vi "Day 2 Puzzle 2.vi"() -> ()   [LabVIEW 2021]
uses:
  <vilib>/Utility/file.llb/Read Delimited Spreadsheet (string).vi
panel:
  out "Sum":i32
  out "Outcomes":i32[](array[numeric])
  in  "Path":path
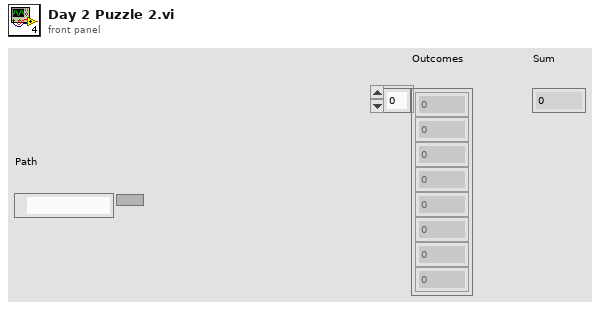
[diagram p1: front panel]
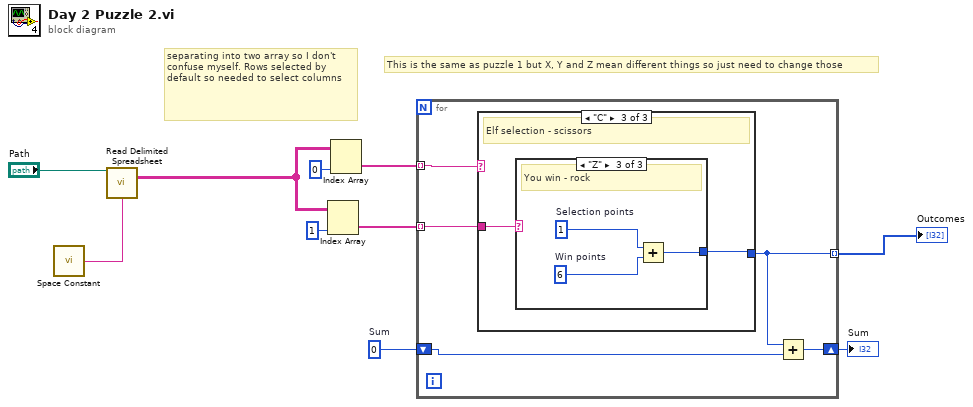
[diagram p0: block diagram]
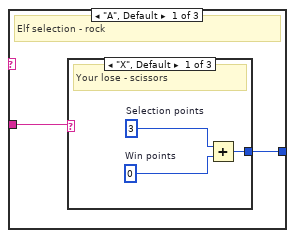
[diagram p2: hidden frame]
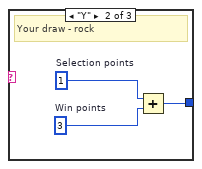
[diagram p3: hidden frame]
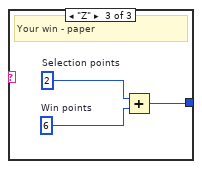
[diagram p4: hidden frame]
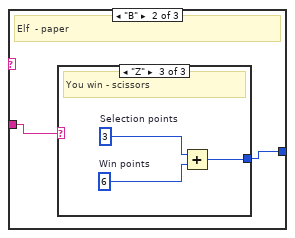
[diagram p5: hidden frame]
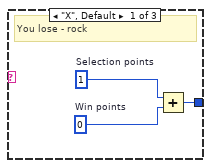
[diagram p6: hidden frame]
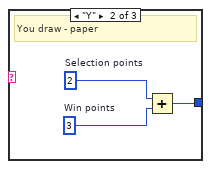
[diagram p7: hidden frame]
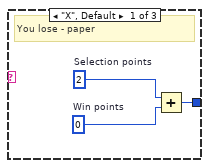
[diagram p8: hidden frame]
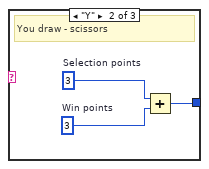
[diagram p9: hidden frame]
diagram:
  w2 = 0  # Sum
  # "This is the same as puzzle 1 but X, Y and Z mean different things so just need to change those"
  # "separating into two array so I don't confuse myself. Rows selected by default so needed to select columns"
  n1 = call <vilib>:"Space Constant.vi"() -> ("String"=w9:string)
  n2 = call-poly <vilib>:"Read Delimited Spreadsheet.vi"("file path (dialog if empty)"="Path", "delimiter (\\t)"=w9) -> ("all rows"=w8:string[][])  [unwired: 8 in, 5 out]
  n3 = Index Array(array=w8, index (col)=1 ("disabled index (col)")) -> (element=w6:string[])  [unwired: 1 in]
  n4 = Index Array(array=w8, index (col)=0 ("disabled index (col)")) -> (element=w7:string[])  [unwired: 1 in]
  n5 = for {
    tunnel: w7 -> [w15] mode=indexing
    tunnel: w6 -> [w14] mode=indexing
    tunnel: [w12] -> w3 mode=indexing
    shift-right: [w13] -> w1
    shift-left: w2 -> [w11]
    n6 = case shown="\"C\"" w15 {
      tunnel: w14 -> [w17 w27 w39]
      tunnel: [w16 w28 w38] -> w12
      frame "A", Default {
        # "Elf selection - rock"
        n7 = case shown="\"X\", Default" w17 {
          tunnel: [w18 w21 w24] -> w16
          frame "X", Default {
            w20 = 0  # Win points
            w19 = 3  # Selection points
            # "Your lose - scissors"
            n8 = Add(x=w19, y=w20) -> (x+y=w18:i32)
          }
          frame "Y" {
            w23 = 3  # Win points
            w22 = 1  # Selection points
            # "Your draw - rock"
            n9 = Add(x=w22, y=w23) -> (x+y=w21:i32)
          }
          frame "Z" {
            w26 = 6  # Win points
            w25 = 2  # Selection points
            # "Your win - paper"
            n10 = Add(x=w25, y=w26) -> (x+y=w24:i32)
          }
        }
      }
      frame "B" {
        # "Elf  - paper"
        n11 = case shown="\"Z\"" w27 {
          tunnel: [w29 w32 w35] -> w28
          frame "X", Default {
            w31 = 0  # Win points
            w30 = 1  # Selection points
            # "You lose - rock"
            n12 = Add(x=w30, y=w31) -> (x+y=w29:i32)
          }
          frame "Y" {
            w34 = 3  # Win points
            w33 = 2  # Selection points
            # "You draw - paper"
            n13 = Add(x=w33, y=w34) -> (x+y=w32:i32)
          }
          frame "Z" {
            w37 = 6  # Win points
            w36 = 3  # Selection points
            # "You win - scissors"
            n14 = Add(x=w36, y=w37) -> (x+y=w35:i32)
          }
        }
      }
      frame "C" {
        # "Elf selection - scissors"
        n15 = case shown="\"Z\"" w39 {
          tunnel: [w40 w43 w46] -> w38
          frame "X", Default {
            w42 = 0  # Win points
            w41 = 2  # Selection points
            # "You lose - paper"
            n16 = Add(x=w41, y=w42) -> (x+y=w40:i32)
          }
          frame "Y" {
            w45 = 3  # Win points
            w44 = 3  # Selection points
            # "You draw - scissors"
            n17 = Add(x=w44, y=w45) -> (x+y=w43:i32)
          }
          frame "Z" {
            w48 = 6  # Win points
            w47 = 1  # Selection points
            # "You win - rock"
            n18 = Add(x=w47, y=w48) -> (x+y=w46:i32)
          }
        }
      }
    }
    n19 = Add(x=w12, y=w11) -> (x+y=w13:i32)
  }
  "Outcomes" <- w3
  "Sum" <- w1
